vi "SetObjectData.vi"(0 "real object ref":refnum<class "G#Object.lvclass">, 5 "error in (no error)":errorcluster) -> (14 "remote ref":refnum<class "G#Object.lvclass">, 19 "error out":errorcluster)   [LabVIEW 2017, in "G#DebugServer.lvclass"]
doc: "Reads the object data and stores it in the native attributes."
uses:
  G#DebugServer.lvclass
  G#Object/G#Object.lvclass
  C:/Program Files (x86)/National Instruments/LabVIEW 2017/vi.lib/addons/_AddQ/G#Object/G#Object.lvclass
  G#DebugServer.lvclass/G#DebugServer.ctl
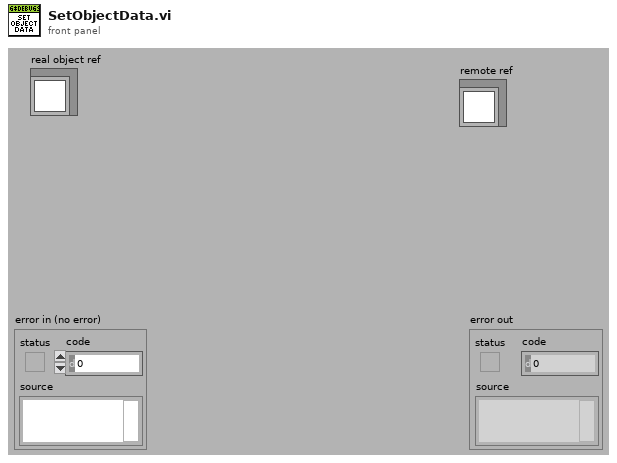
[diagram p1: front panel]
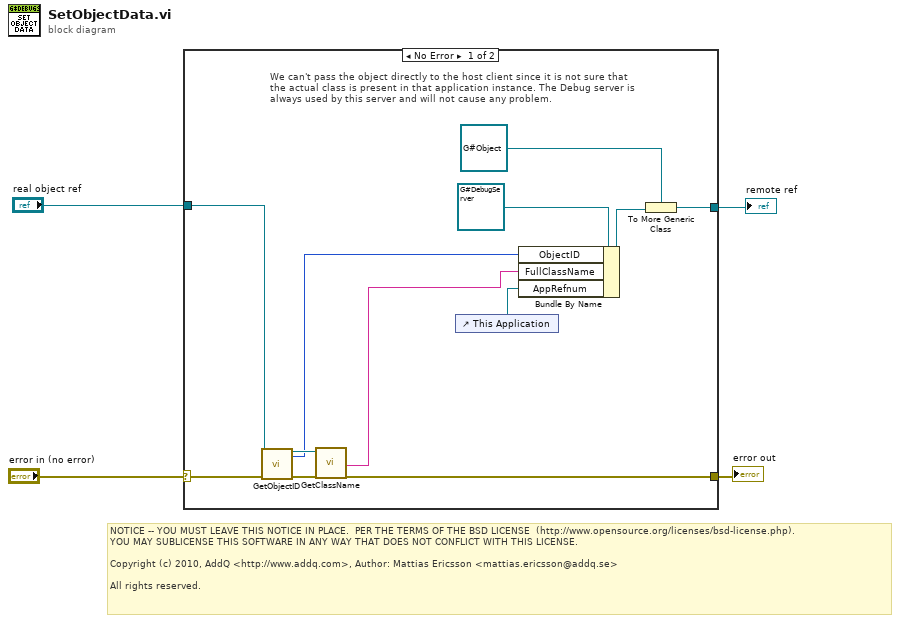
[diagram p0: block diagram]
diagram:
  # "NOTICE -- YOU MUST LEAVE THIS NOTICE IN PLACE.  PER THE TERMS OF THE BSD LICENSE  (http://www.opensource.org/licenses/bsd-license.php).\nYOU MAY SUBLICENSE THIS SOFTWARE IN ANY WAY THAT DOES NOT CONFLICT WITH THIS LICENSE.\n\nCopyright (c) 2010, AddQ <http://www.addq.com>, Author: Mattias Ericsson <mattias.ericsson@addq.se>\n\nAll rights reserved."
  n1 = case shown="No Error" "error in (no error)" {
    selector: "error in (no error)" -> [w16 w18]
    tunnel: [w14 w18] -> w3
    tunnel: "real object ref" -> [w10 w17]
    tunnel: [w8 w17] -> w1
    frame No Error {
      # "We can't pass the object directly to the host client since it is not sure that\nthe actual class is present in that application instance. The Debug server is\nalways used by this server and will not cause any problem."
      n2 = call-dynamic "GetObjectID.vi"("reference in"=w10, "error in (no error)"=w16) -> ("reference out"=w13:refnum<class "G#Object.lvclass">, "object ID"=w12:u32, "error out"=w15:errorcluster)  [unwired: 15 in]
      n3 = call-dynamic "GetClassName.vi"("reference in"=w13, "error in (no error)"=w15) -> ("full class name"=w11:string, "error out"=w14:errorcluster)  [unwired: 13 in, 3 out]
      n4 = control-ref of="This Application"() -> (w6:refnum<vi>)
      n5 = Bundle By Name(cluster=refnum<class "G#DebugServer.lvclass"> refnum ("G#DebugServer reference out"), "ObjectID"=w12, "FullClassName"=w11, "AppRefnum"=w6) -> (w5:refnum<class "G#DebugServer.lvclass">)
      n6 = To More Generic Class(target class=refnum<class "G#Object.lvclass"> refnum ("G#Object reference in"), reference=w5) -> (generic class reference=w8:refnum<class "G#Object.lvclass">)
    }
    frame Error {
    }
  }
  "error out" <- w3
  "remote ref" <- w1
